vi "子VI-修改评定结果.vi"(9 "全部检测结果":string[][](table), 11 "临界面积百分比值":dbl) -> (1 "全部检测结果合并输出":string[][](table) caption="全部检测结果")   [LabVIEW 2018]
panel:
  in  "ok":bool
  in  "确定按钮":bool
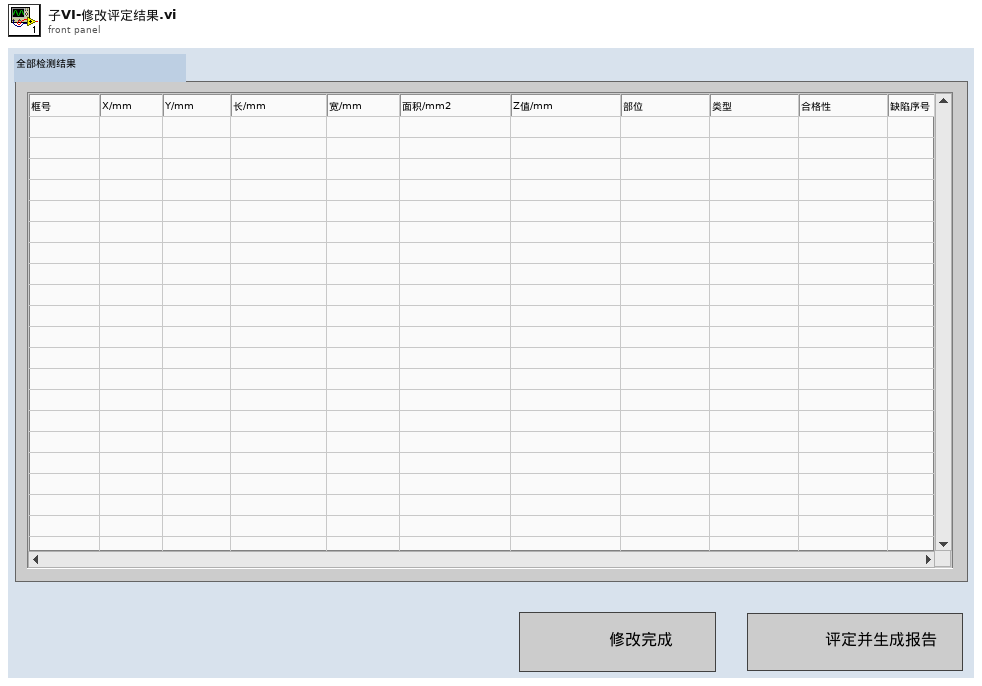
[diagram p1: front panel]
types:
  T1 = enum8{"Enabled", "Disabled", "Disabled and Grayed Out"}
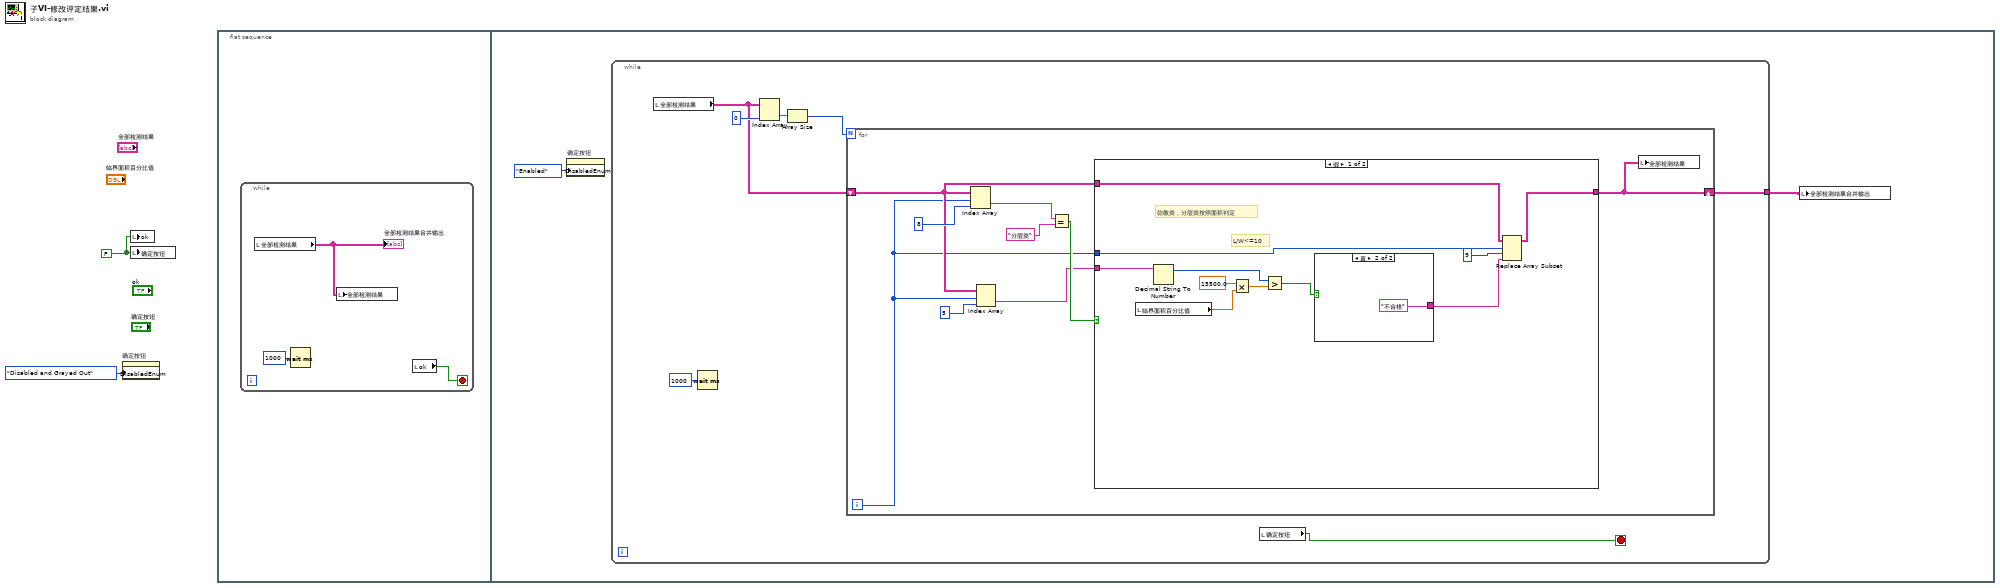
[diagram p0: block diagram]
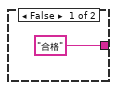
[diagram p2: hidden frame]
diagram:
  w2 = FALSE
  n1 = property on="确定按钮" class="Bool (严格)"("DisabledEnum"=T1."Disabled and Grayed Out" ("禁用")) -> ()  [unwired: 2 in, 2 out]
  n2 = local write "ok"(w2) -> ()
  n3 = local write "确定按钮"(w2) -> ()
  n4 = flat-sequence {
    frame #0 {
      n5 = while {
        stop <- w3 stop-if-true
        n6 = local read "全部检测结果"() -> (w4:string[][])
        "全部检测结果合并输出" <- w4
        n7 = Wait (ms)(milliseconds to wait=u32 1000 ("等待时间（毫秒）")) -> ()  [unwired: 1 out]
        n8 = local write "全部检测结果"(w4) -> ()
        n9 = local read "ok"() -> (w3:bool)
      }
    }
    frame #1 {
      n10 = property on="确定按钮" class="Bool (严格)"("DisabledEnum"=T1."Enabled" ("禁用")) -> ()  [unwired: 2 in, 2 out]
      n11 = while {
        tunnel: [w9] -> w6
        stop <- w13 stop-if-true
        n12 = local read "全部检测结果"() -> (w10:string[][])
        n13 = Wait (ms)(milliseconds to wait=u32 1000 ("等待时间（毫秒）")) -> ()  [unwired: 1 out]
        n14 = Index Array(array=w10, index (col)=0 ("禁用的索引 (列)")) -> (element=w11:string[])  [unwired: 1 in]
        n15 = Array Size(array=w11) -> (size(s)=w14:i32)
        n16 = for {
          N: w14 -> [_]
          shift-right: [w15] -> w9
          shift-left: w10 -> [w19]
          i -> [w18]
          n17 = Index Array(array=w19, index (row)=w18, index (col)=8 ("禁用的索引 (列)")) -> (element=w21:string)
          n18 = Index Array(array=w19, index (row)=w18, index (col)=5 ("禁用的索引 (列)")) -> (element=w16:string)
          n19 = Equal?(x=w21, y="分层类") -> (x = y?=w20:bool)
          n20 = case shown="假" w20 {
            tunnel: w19 -> [w31 w37]
            tunnel: w18 -> [w30 _]
            tunnel: [w27 w37] -> w15
            tunnel: w16 -> [w25 _]
            frame False {
              # "L/W<=10"
              # "弥散类，分层类按照面积判定"
              n21 = local read "临界面积百分比值"() -> (w32:dbl)
              n22 = Decimal String To Number(string=w25) -> (offset past number=w24:i32)  [unwired: 2 in, 1 out]
              n23 = Multiply(x=15500.0, y=w32) -> (x*y=w34:dbl)
              n24 = Greater?(x=w24, y=w34) -> (0:w26:bool)
              n25 = case shown="真" w26 {
                tunnel: ["合格" "不合格"] -> w28
                frame False {
                }
                frame True {
                }
              }
              n26 = Replace Array Subset(array=w31, new element=w28, index (row)=w30, index (col)=9 ("禁用的索引 (列)")) -> (w27:string[][])
            }
            frame True {
              # "分层类，合格性按照Z值\n默认不变"
            }
          }
          n27 = local write "全部检测结果"(w15) -> ()
        }
        n28 = local read "确定按钮"() -> (w13:bool)
      }
      n29 = local write "全部检测结果合并输出"(w6) -> ()
    }
  }
